vi "FTW-Message-Initialize.vi"(0 "Message":refnum<class "FTW-Message.lvclass">, 11 "error in":errorcluster) -> (4 "Message out":refnum<class "FTW-Message.lvclass">, 15 "error out":errorcluster)   [LabVIEW 2012, in "FTW-Message.lvclass"]
uses:
  FTW-Message.lvclass
  FTW-Message.lvclass/FTW-Message.ctl
panel:
  # "Inputs"
  # "Outputs"
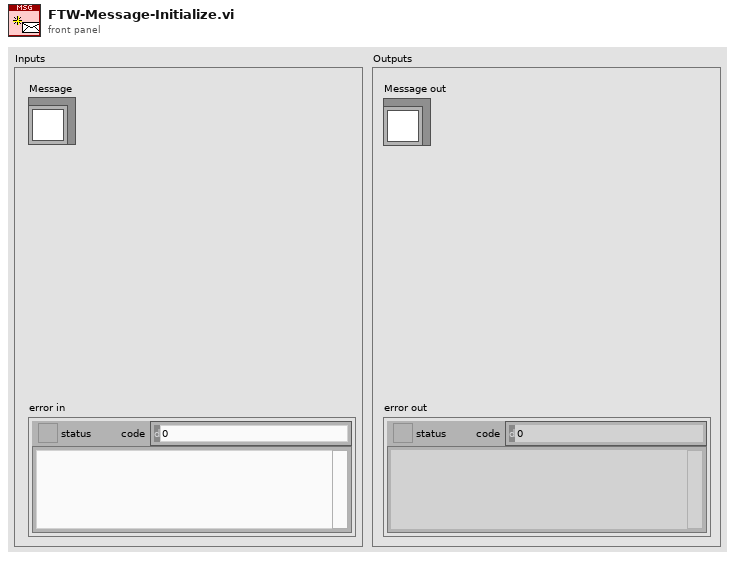
[diagram p1: front panel]
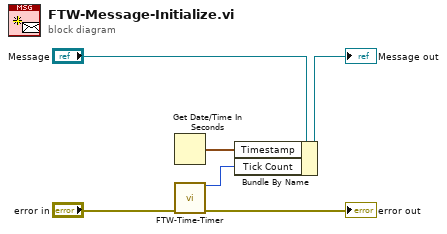
[diagram p0: block diagram]
diagram:
  n1 = Get Date/Time In Seconds() -> (seconds since 1Jan1904=w4:timestamp)
  n2 = call "FTW-Time-Timer.vi"("error in"="error in") -> ("Current Tick Count"=w1:u32, "error out"=→"error out":errorcluster)  [unwired: 12 in, 1 out]
  n3 = Bundle By Name(cluster="Message", "Timestamp"=w4, "Tick Count"=w1) -> (→"Message out":refnum<class "FTW-Message.lvclass">)
